vi "save_data (SubVI).vi"(4 "Process list":T2, 5 "encoded_bits":bool[](array[boolean]), 6 "DC volts arr":dbl[](array[numeric]), 7 "environ cluster":cluster{dbl[], dbl[]}, 8 "imgrid":bool=TRUE, 9 "Sample rate":dbl format="%#_13g", 10 "file_path_cluster":T1, 11 "data":i16[][](array[numeric])) -> ()   [LabVIEW 2014]
uses:
  <vilib>/addons/h5labview2/file/H5Fmode.ctl
  <vilib>/addons/h5labview2/base/lib_path.vi
  <vilib>/addons/h5labview2/base/H5Equery.vi
  <vilib>/addons/h5labview2/dataset/H5Dwrite.llb/H5Dwrite.xnode
  <vilib>/addons/h5labview2/attrib/H5Awrite.llb/H5Awrite.xnode
  <vilib>/addons/h5labview2/base/hid_t.ctl
  <vilib>/addons/h5labview2/file/H5F.lvlib
  <vilib>/addons/h5labview2/group/H5G.lvlib
  National Instruments Downloads/LabVIEW FPGA English/FPGA Timekeeper 1.1b0/FPGA Timekeeper.lvlib
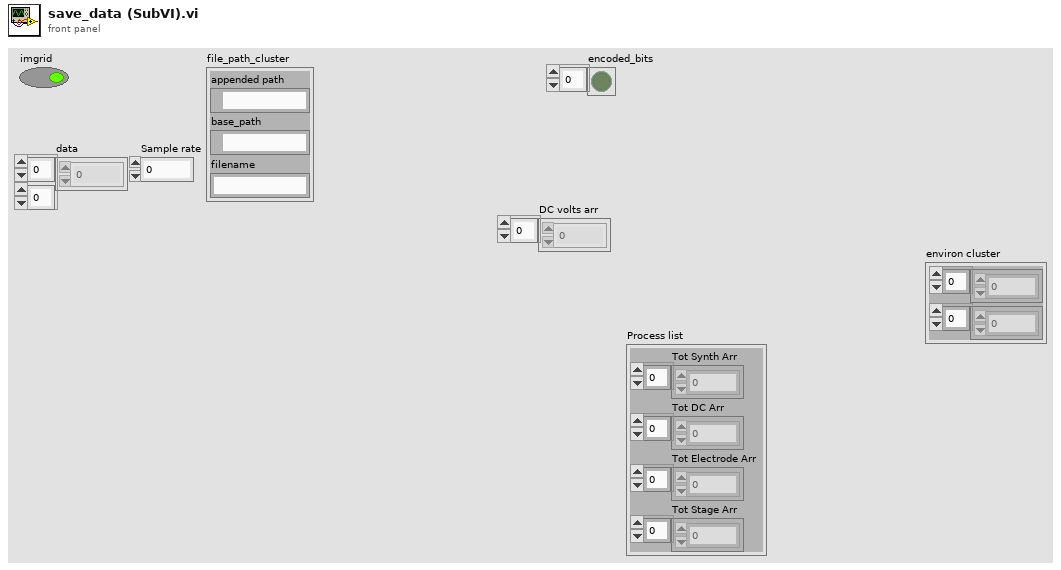
[diagram p1: front panel]
types:
  T1 = cluster{"appended path":path, "base_path":path, "filename":string}
  T2 = cluster{"Tot Synth Arr":dbl[], "Tot DC Arr":dbl[], "Tot Electrode Arr":dbl[], "Tot Stage Arr":dbl[]}
  T3 = typedef "H5F.lvlib/H5Fmode.ctl" = enum16{"read-only", "read-write", "overwrite", "create new", "open or create"}
  T4 = typedef "hid_t.ctl" = i32
  T5 = cluster{"Sample rate":dbl, dbl, dbl[], dbl[], "Tot Synth Arr":dbl[], "Tot DC Arr":dbl[], "Tot Electrode Arr":dbl[], "DC volts arr":dbl[], "Tot Stage Arr":dbl[], "encoded_bits":bool[], "imgrid":bool}
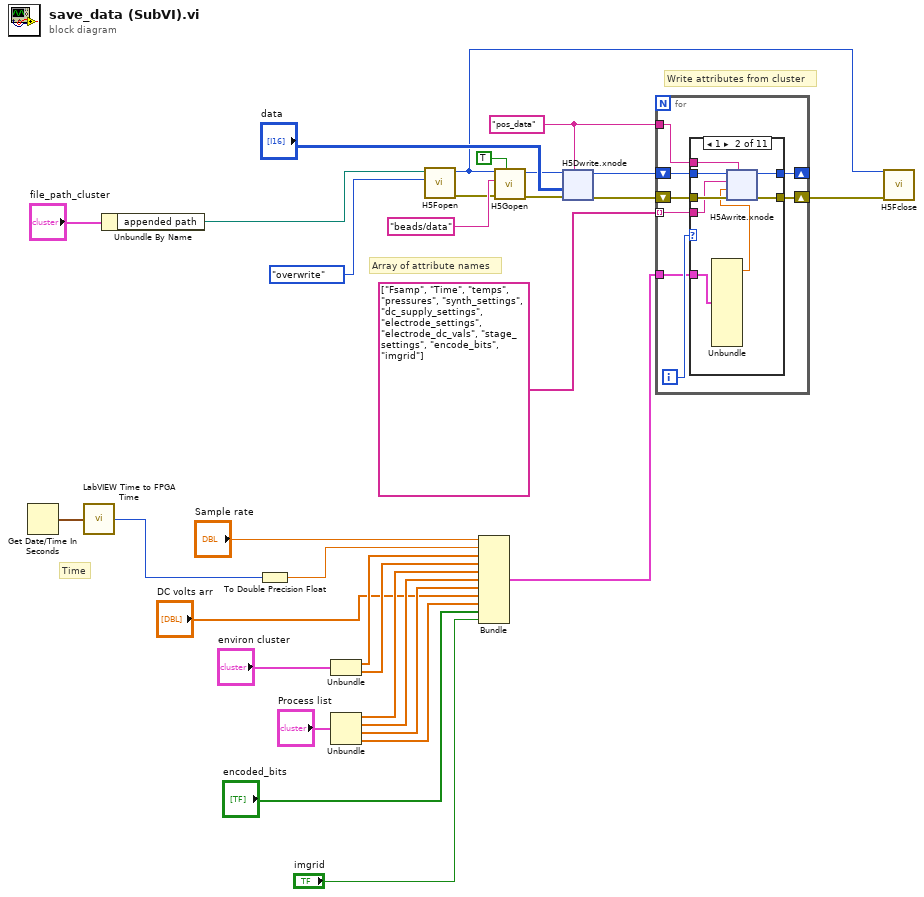
[diagram p0: block diagram]
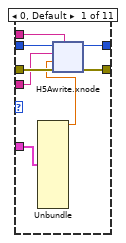
[diagram p2: hidden frame]
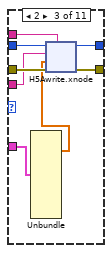
[diagram p3: hidden frame]
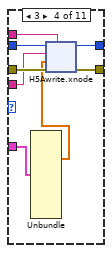
[diagram p4: hidden frame]
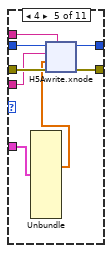
[diagram p5: hidden frame]
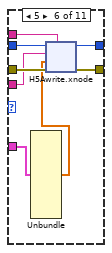
[diagram p6: hidden frame]
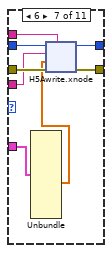
[diagram p7: hidden frame]
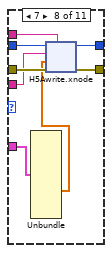
[diagram p8: hidden frame]
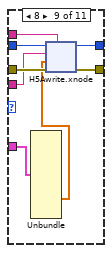
[diagram p9: hidden frame]
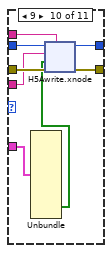
[diagram p10: hidden frame]
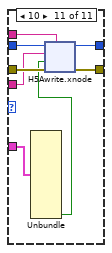
[diagram p11: hidden frame]
diagram:
  w31 = "pos_data" ("dataset name")
  # "Time"
  # "Array of attribute names"
  # "Write attributes from cluster"
  n1 = Get Date/Time In Seconds() -> (seconds since 1Jan1904=w3:timestamp)
  n2 = call "LabVIEW Time to FPGA Time.vi"("LabVIEW time"=w3) -> ("FPGA time (ns)"=w1:u64)
  n3 = Unbundle By Name("file_path_cluster") -> ("appended path"=w6:path)
  n4 = To Double Precision Float(number=w1) -> (double precision float=w2:dbl)
  n5 = Unbundle("environ cluster") -> (w18:dbl[], w17:dbl[])
  n6 = Unbundle("Process list") -> ("Tot Synth Arr"=w12:dbl[], "Tot DC Arr"=w11:dbl[], "Tot Electrode Arr"=w10:dbl[], "Tot Stage Arr"=w9:dbl[])
  n7 = call <vilib>:"H5Fopen.vi"("mode (read-only)"=H5Fmode."overwrite", "path"=w6) -> ("error out"=w24:errorcluster, "ref out"=w14:T4)  [unwired: 8 in]
  n8 = Bundle("Sample rate"="Sample rate", w2, w18, w17, "Tot Synth Arr"=w12, "Tot DC Arr"=w11, "Tot Electrode Arr"=w10, "DC volts arr"="DC volts arr", "Tot Stage Arr"=w9, "encoded_bits"="encoded_bits", "imgrid"="imgrid") -> (w16:T5)  [unwired: 1 in]
  n9 = call <vilib>:"H5Gopen.vi"("create? (F)"=TRUE, "error in (no error)"=w24, "name"="beads/data", "ref in"=w14) -> ("error out"=w29:errorcluster, "group out"=w15:T4)  [unwired: 6 in]
  n10 = xnode "H5Dwrite.xnode"("dataset name"=w31, "error in (no error)"=w29, "data"="data", "ref in"=w15) -> ("error out"=w28:errorcluster, "ref out"=w22:i32)  [unwired: 3 in, 1 out]
  n11 = for {
    tunnel: w31 -> [w39]
    shift-right: [w37] -> _
    shift-left: w22 -> [w34]
    shift-right: [w36] -> w26
    shift-left: w28 -> [w38]
    tunnel: string[] ["Fsamp", "Time", "temps", "pressures", "synth_settings", "dc_supply_settings", "electrode_settings", "electrode_dc_vals", "stage_settings", "encode_bits", "imgrid"] -> [w35] mode=indexing
    tunnel: w16 -> [w32]
    i -> [w33]
    n12 = case shown="1" w33 {
      tunnel: w39 -> [w47 w73 w99 w125 w151 w177 w203 w229 w255 w281 w307]
      tunnel: w38 -> [w46 w72 w98 w124 w150 w176 w202 w228 w254 w279 w305]
      tunnel: [w45 w71 w97 w123 w149 w175 w201 w227 w253 w276 w303] -> w37
      tunnel: [w44 w70 w96 w122 w148 w174 w200 w226 w252 w275 w302] -> w36
      tunnel: w35 -> [w43 w69 w95 w121 w147 w173 w199 w225 w251 w274 w301]
      tunnel: w34 -> [w42 w68 w94 w120 w146 w172 w198 w224 w250 w280 w306]
      tunnel: w32 -> [w41 w67 w93 w119 w145 w171 w197 w223 w249 w278 w304]
      frame 0, Default {
        n13 = Unbundle(w41) -> ("Sample rate"=w40:dbl)  [unwired: 10 out]
        n14 = xnode "H5Awrite.xnode"("object name"=w47, "error in (no error)"=w46, "data"=w40, "attrib name"=w43, "ref in"=w42) -> ("error out"=w44:errorcluster, "ref out"=w45:T4)  [unwired: 2 in, 1 out]
      }
      frame 1 {
        n15 = Unbundle(w67) -> (w66:dbl)  [unwired: 10 out]
        n16 = xnode "H5Awrite.xnode"("object name"=w73, "error in (no error)"=w72, "data"=w66, "attrib name"=w69, "ref in"=w68) -> ("error out"=w70:errorcluster, "ref out"=w71:T4)  [unwired: 2 in, 1 out]
      }
      frame 2 {
        n17 = Unbundle(w93) -> (w92:dbl[])  [unwired: 10 out]
        n18 = xnode "H5Awrite.xnode"("object name"=w99, "error in (no error)"=w98, "data"=w92, "attrib name"=w95, "ref in"=w94) -> ("error out"=w96:errorcluster, "ref out"=w97:T4)  [unwired: 2 in, 1 out]
      }
      frame 3 {
        n19 = Unbundle(w119) -> (w118:dbl[])  [unwired: 10 out]
        n20 = xnode "H5Awrite.xnode"("object name"=w125, "error in (no error)"=w124, "data"=w118, "attrib name"=w121, "ref in"=w120) -> ("error out"=w122:errorcluster, "ref out"=w123:T4)  [unwired: 2 in, 1 out]
      }
      frame 4 {
        n21 = Unbundle(w145) -> ("Tot Synth Arr"=w144:dbl[])  [unwired: 10 out]
        n22 = xnode "H5Awrite.xnode"("object name"=w151, "error in (no error)"=w150, "data"=w144, "attrib name"=w147, "ref in"=w146) -> ("error out"=w148:errorcluster, "ref out"=w149:T4)  [unwired: 2 in, 1 out]
      }
      frame 5 {
        n23 = Unbundle(w171) -> ("Tot DC Arr"=w170:dbl[])  [unwired: 10 out]
        n24 = xnode "H5Awrite.xnode"("object name"=w177, "error in (no error)"=w176, "data"=w170, "attrib name"=w173, "ref in"=w172) -> ("error out"=w174:errorcluster, "ref out"=w175:T4)  [unwired: 2 in, 1 out]
      }
      frame 6 {
        n25 = Unbundle(w197) -> ("Tot Electrode Arr"=w196:dbl[])  [unwired: 10 out]
        n26 = xnode "H5Awrite.xnode"("object name"=w203, "error in (no error)"=w202, "data"=w196, "attrib name"=w199, "ref in"=w198) -> ("error out"=w200:errorcluster, "ref out"=w201:T4)  [unwired: 2 in, 1 out]
      }
      frame 7 {
        n27 = Unbundle(w223) -> ("DC volts arr"=w222:dbl[])  [unwired: 10 out]
        n28 = xnode "H5Awrite.xnode"("object name"=w229, "error in (no error)"=w228, "data"=w222, "attrib name"=w225, "ref in"=w224) -> ("error out"=w226:errorcluster, "ref out"=w227:T4)  [unwired: 2 in, 1 out]
      }
      frame 8 {
        n29 = Unbundle(w249) -> ("Tot Stage Arr"=w248:dbl[])  [unwired: 10 out]
        n30 = xnode "H5Awrite.xnode"("object name"=w255, "error in (no error)"=w254, "data"=w248, "attrib name"=w251, "ref in"=w250) -> ("error out"=w252:errorcluster, "ref out"=w253:T4)  [unwired: 2 in, 1 out]
      }
      frame 9 {
        n31 = Unbundle(w278) -> ("encoded_bits"=w277:bool[])  [unwired: 10 out]
        n32 = xnode "H5Awrite.xnode"("object name"=w281, "error in (no error)"=w279, "data"=w277, "attrib name"=w274, "ref in"=w280) -> ("error out"=w275:errorcluster, "ref out"=w276:T4)  [unwired: 2 in, 1 out]
      }
      frame 10 {
        n33 = Unbundle(w304) -> ("imgrid"=w300:bool)  [unwired: 10 out]
        n34 = xnode "H5Awrite.xnode"("object name"=w307, "error in (no error)"=w305, "data"=w300, "attrib name"=w301, "ref in"=w306) -> ("error out"=w302:errorcluster, "ref out"=w303:T4)  [unwired: 2 in, 1 out]
      }
    }
  }
  n35 = call <vilib>:"H5Fclose.vi"("error in (no error)"=w26, "ref"=w14) -> ()  [unwired: 9 in, 1 out]
